vi "Read Response.vi"(8 "error in":errorcluster, 11 "ThorlabsLabJack in":refnum<class "ThorlabsLabJack.lvclass">) -> (0 "error out":errorcluster, 2 "Success?":bool, 3 "ThorlabsLabJack out":refnum<class "ThorlabsLabJack.lvclass">)   [LabVIEW 2018, in "ThorlabsLabJack.lvlib" / "ThorlabsLabJack.lvclass"]
doc: "This VI is used in conjunction with Send Command. Send Command, when using certain types, will send a command to the instrument. Read Response will read the response to make sure the command was valid. Success will be true if the last command was valid."
uses:
  ThorlabsLabJack.lvclass
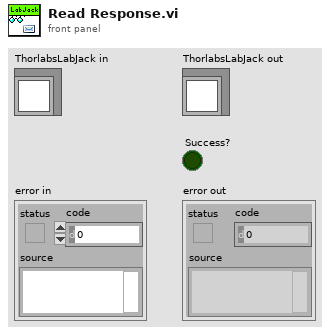
[diagram p1: front panel]
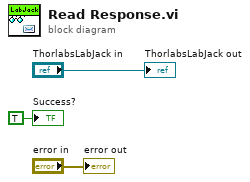
[diagram p0: block diagram]
diagram:
  "error out" <- "error in"
  "ThorlabsLabJack out" <- "ThorlabsLabJack in"
  "Success?" <- TRUE ("Success?")
